vi "key_bind.vi"(10 "keyboard bind":string, 11 "current char in":i16) -> (3 "output value (note)":bool, 6 "current char out":i16)   [LabVIEW 2024]
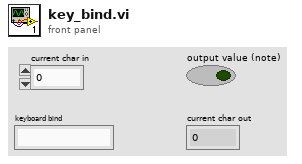
[diagram p1: front panel]
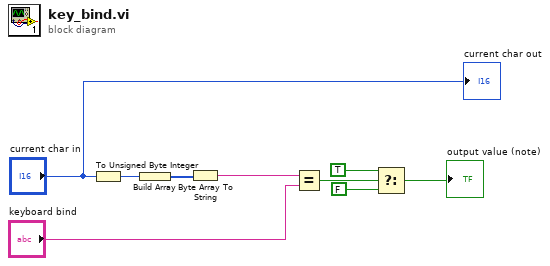
[diagram p0: block diagram]
diagram:
  n1 = To Unsigned Byte Integer(number="current char in") -> (unsigned 8bit integer=w9:u8)
  n2 = Build Array(w9) -> (w8:u8[])
  n3 = Byte Array To String(unsigned byte array=w8) -> (string=w7:string)
  n4 = Equal?(x=w7, y="keyboard bind") -> (x = y?=w2:bool)
  n5 = Select(t=TRUE, s=w2, f=FALSE) -> (s? t:f=→"output value (note)":bool)
  "current char out" <- "current char in"
